vi "Single SSC Relay NI-Switch Control.vi"(0 "SSC Relay in":T1, 7 "Operation":T2=21 items=["Open Relay"=20, "Close Relay"=21], 11 "error in":errorcluster) -> (3 "Completed Relay Operations":T3 {"Desired State" items=["Open Relay"=20, "Close Relay"=21]}, 4 "SSC Relay out":T1, 15 "error out":errorcluster)   [LabVIEW 2019]
doc: "This VI executes the NI-Switch driver to perform the specified relay operation on the Relay channel contained within the Relay SSC input. If the relay was already in the position that was requested by the operation, no operation will be performed."
uses:
  SubVIs/TSM Relay Completed Operations.ctl
  <instrlib>/niSwitch/niSwitch.llb/niSwitch Relay Action.ctl
  SSC Relay.ctl
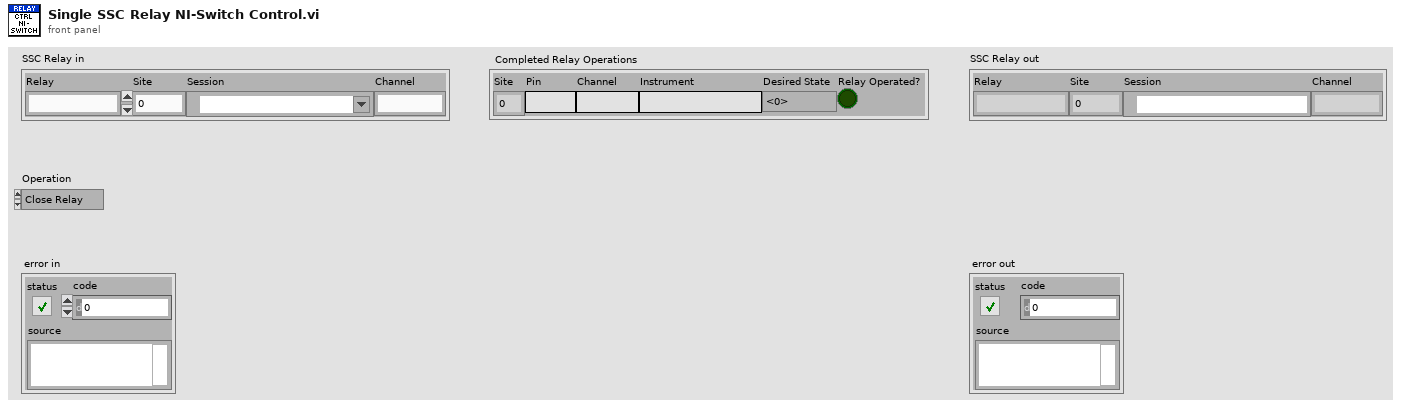
[diagram p1: front panel]
types:
  T1 = typedef "SSC Relay.ctl" = cluster{"Relay":string, "Site":i32, "Session":refnum<k15>, "Channel":string}
  T2 = typedef "niSwitch Relay Action.ctl" = i32
  T3 = typedef "TSM Relay Completed Operations.ctl" = cluster{"Site":i32, "Pin":string, "Channel":string, "Instrument":string, "Desired State":T2, "Relay Operated?":bool}
  T4 = typedef "niSwitch Relay Position.ctl" = i32
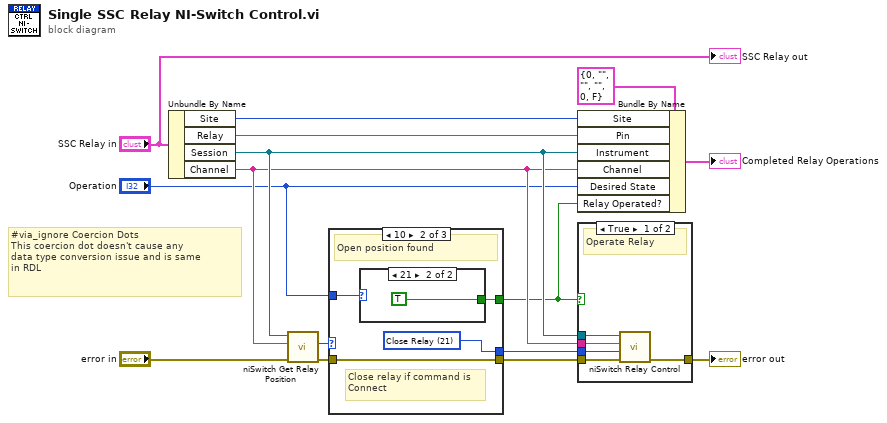
[diagram p0: block diagram]
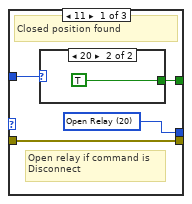
[diagram p2: hidden frame]
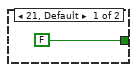
[diagram p3: hidden frame]
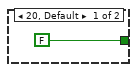
[diagram p4: hidden frame]
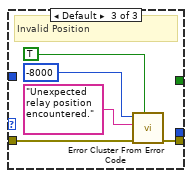
[diagram p5: hidden frame]
diagram:
  # "#via_ignore Coercion Dots\nThis coercion dot doesn't cause any\ndata type conversion issue and is same\nin RDL"
  n1 = Unbundle By Name("SSC Relay in") -> ("Site"=w4:i32, "Relay"=w5:string, "Session"=w15:refnum<k15>, "Channel"=w6:string)
  n2 = call <instrlib>:"niSwitch Get Relay Position.vi"("error in (no error)"="error in", "relay name"=w6, "instrument handle"=w15) -> ("error out"=w10:errorcluster, "position"=w9:T4)  [unwired: 6 in, 1 out]
  n3 = case shown="10" w9 {
    tunnel: w10 -> [w19 w25 w30]
    tunnel: [w19 w25 w29] -> w11
    tunnel: [w16 w23 _] -> w1
    tunnel: "Operation" -> [w17 w24 _]
    tunnel: [w18 w22 _] -> w8
    frame 11 {
      w18 = T2 20 items=["Open Relay"=20, "Close Relay"=21] ("relay action (Close Relay)")
      # "Open relay if command is\nDisconnect"
      # "Closed position found"
      n4 = case shown="20" w17 {
        tunnel: [FALSE TRUE] -> w16
        frame 21, Default {
        }
        frame 20 {
        }
      }
    }
    frame 10 {
      w22 = T2 21 items=["Open Relay"=20, "Close Relay"=21] ("relay action (Close Relay)")
      # "Close relay if command is\nConnect"
      # "Open position found"
      n5 = case shown="21" w24 {
        tunnel: [FALSE TRUE] -> w23
        frame 20, Default {
        }
        frame 21 {
        }
      }
    }
    frame Default {
      # "Invalid Position"
      n6 = call <vilib>:"Error Cluster From Error Code.vi"("show call chain? (False)"=TRUE, "error in (no error)"=w30, "error message (\"\")"="Unexpected relay position encountered." ("error message (\"\")"), "error code (0)"=-8000) -> ("error out"=w29:errorcluster)  [unwired: 5 in]
    }
  }
  n7 = Bundle By Name(cluster=T3 {"Site"=0, "Pin"="", "Channel"="", "Instrument"="", "Desired State"=0, "Relay Operated?"=FALSE} ("Relay - Switch Operations Completed"), "Site"=w4, "Pin"=w5, "Instrument"=w15, "Channel"=w6, "Desired State"="Operation", "Relay Operated?"=w1) -> (→"Completed Relay Operations":T3)
  n8 = case shown="True" w1 {
    tunnel: w11 -> [w37 w38]
    tunnel: w6 -> [w34 _]
    tunnel: [w36 w38] -> w13
    tunnel: w15 -> [w35 _]
    tunnel: w8 -> [w33 _]
    frame True {
      # "Operate Relay"
      n9 = call <instrlib>:"niSwitch Relay Control.vi"("error in (no error)"=w37, "relay action (Close Relay)"=w33, "relay names"=w34, "instrument handle"=w35) -> ("error out"=w36:errorcluster)  [unwired: 6 in, 1 out]
    }
    frame False {
      # "No Change"
    }
  }
  "error out" <- w13
  "SSC Relay out" <- "SSC Relay in"
